vi "Stack Images.vi"(8 "Padding":u8, 9 "Vertical?":bool=TRUE, 10 "BG Color":u32(colorbox)=16777215, 11 "Array":picture[](array[picture])) -> (3 "empty picture":picture)   [LabVIEW 2016]
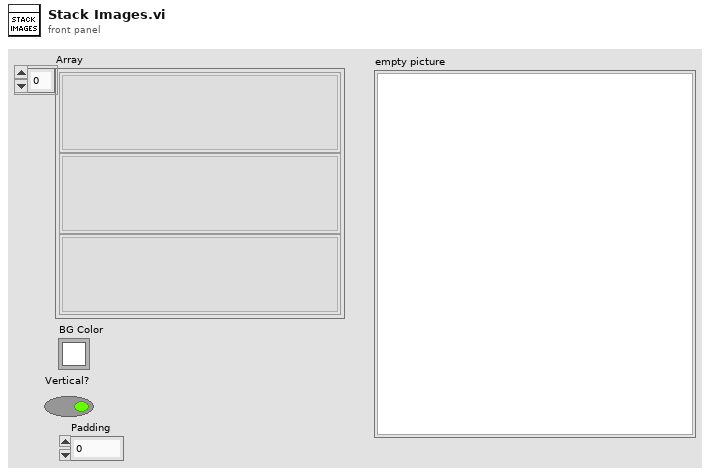
[diagram p1: front panel]
types:
  T1 = cluster{"left":i16, "top":i16, "right":i16, "bottom":i16}
  T2 = typedef "imagedata.ctl" = cluster{"image type":i32, "image depth":i32, "image":u8[], "mask":u8[], "colors":u32[], "Rectangle":cluster{"left":i16, "top":i16, "right":i16, "bottom":i16}}
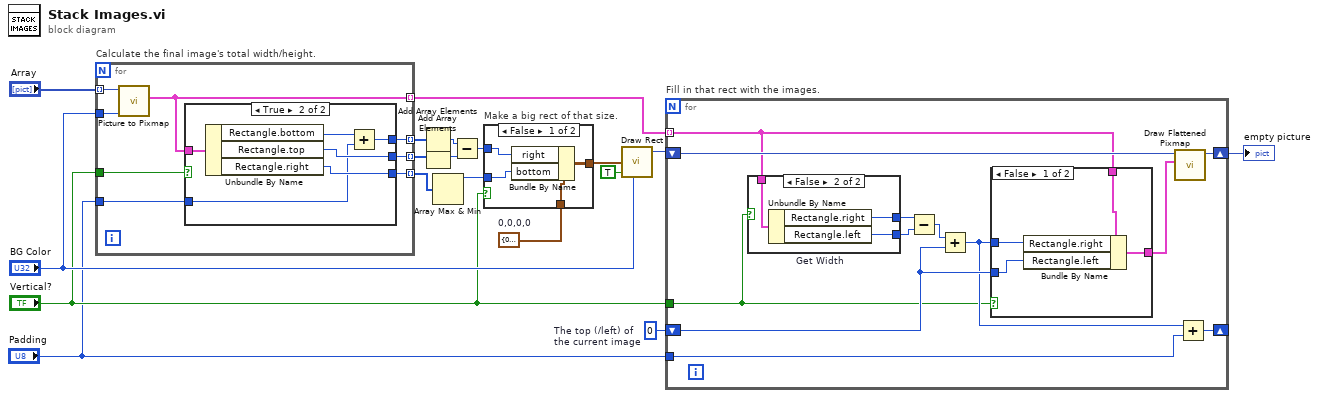
[diagram p0: block diagram]
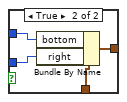
[diagram p2: hidden frame]
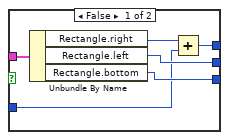
[diagram p3: hidden frame]
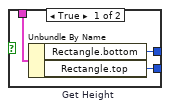
[diagram p4: hidden frame]
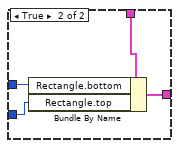
[diagram p5: hidden frame]
diagram:
  w4 = i16 0  # The top (/left) of the current image
  w13 = T1 {"left"=0, "top"=0, "right"=0, "bottom"=0}  # 0,0,0,0
  n1 = for "Calculate the final image's total width/height." {
    tunnel: "Array" -> [w26] mode=indexing
    tunnel: [w25] -> w7 mode=indexing
    tunnel: [w24] -> w6 mode=indexing
    tunnel: [w23] -> w5 mode=indexing
    tunnel: [w22] -> w14 mode=indexing
    tunnel: "BG Color" -> [w21]
    tunnel: "Vertical?" -> [w20]
    tunnel: "Padding" -> [w19]
    n2 = call <vilib>:"Picture to Pixmap.vi"("Background Color"=w21, "picture"=w26) -> ("image data"=w25:T2)  [unwired: 8 in, 1 out]
    n3 = case shown="True" w20 {
      tunnel: w25 -> [w32 w38]
      tunnel: [w30 w36] -> w24
      tunnel: [w29 w35] -> w23
      tunnel: [w28 w34] -> w22
      tunnel: w19 -> [w27 w33]
      frame False {
        n4 = Unbundle By Name(w32) -> ("Rectangle.right"=w31:i16, "Rectangle.left"=w29:i16, "Rectangle.bottom"=w28:i16)
        n5 = Add(x=w31, y=w27) -> (x+y=w30:i16)
      }
      frame True {
        n6 = Unbundle By Name(w38) -> ("Rectangle.bottom"=w37:i16, "Rectangle.top"=w35:i16, "Rectangle.right"=w34:i16)
        n7 = Add(x=w37, y=w33) -> (x+y=w36:i16)
      }
    }
  }
  n8 = Add Array Elements(numeric array=w6) -> (sum=w15:i16)
  n9 = Add Array Elements(numeric array=w5) -> (sum=w16:i16)
  n10 = Array Max & Min(array=w14) -> (max value=w11:i16)  [unwired: 3 out]
  n11 = Subtract(x=w15, y=w16) -> (x-y=w12:i16)
  n12 = case "Make a big rect of that size." shown="False" "Vertical?" {
    tunnel: w13 -> [w42 w46]
    tunnel: w12 -> [w40 w43]
    tunnel: w11 -> [w39 w44]
    tunnel: [w41 w45] -> w10
    frame False {
      n13 = Bundle By Name(cluster=w42, "right"=w40, "bottom"=w39) -> (w41:T1)
    }
    frame True {
      n14 = Bundle By Name(cluster=w46, "bottom"=w43, "right"=w44) -> (w45:T1)
    }
  }
  n15 = call <vilib>:"Draw Rect.vi"("rect"=w10, "fill?(F)"=TRUE, "color(black)"="BG Color") -> ("new picture"=w8:picture)  [unwired: 6 in]
  n16 = for "Fill in that rect with the images." {
    shift-right: [w57] -> w18
    shift-left: w8 -> [w58]
    shift-right: [w49] -> _
    shift-left: w4 -> [w51]
    tunnel: w7 -> [w56] mode=indexing
    tunnel: "Vertical?" -> [w48]
    tunnel: "Padding" -> [w47]
    n17 = case shown="False" w48 {
      tunnel: w56 -> [w61 w64]
      tunnel: [w60 w63] -> w55
      tunnel: [w59 w62] -> w54
      frame True {
        n18 = Unbundle By Name "Get Height"(w61) -> ("Rectangle.bottom"=w60:i16, "Rectangle.top"=w59:i16)
      }
      frame False {
        n19 = Unbundle By Name "Get Width"(w64) -> ("Rectangle.right"=w63:i16, "Rectangle.left"=w62:i16)
      }
    }
    n20 = Subtract ("Height")(x=w55, y=w54) -> (x-y=w53:i16)
    n21 = Add(x=w53, y=w51) -> (x+y=w50:i16)
    n22 = case shown="False" w48 {
      tunnel: w56 -> [w67 w71]
      tunnel: w50 -> [w68 w72]
      tunnel: w51 -> [w66 w70]
      tunnel: [w65 w69] -> w52
      frame False {
        n23 = Bundle By Name(cluster=w67, "Rectangle.right"=w68, "Rectangle.left"=w66) -> (w65:T2)
      }
      frame True {
        n24 = Bundle By Name(cluster=w71, "Rectangle.bottom"=w72, "Rectangle.top"=w70) -> (w69:T2)
      }
    }
    n25 = call <vilib>:"Draw Flattened Pixmap.vi"("image data"=w52, "picture"=w58) -> ("new picture"=w57:picture)  [unwired: 7 in]
    n26 = Add(x=w50, y=w47) -> (x+y=w49:i16)
  }
  "empty picture" <- w18
